vi "Combination_Digitizer_Driver_CLEANUP.vi"(0 "Mode":T1(ring), 1 "Horizontal Settings":T2={"number of records"=1, "reference position"=50.0, "min record length"=50000, "min sample rate"=200000.0, "enforce realtime"=FALSE, "maximum input frequency"=0.0} {"maximum input frequency" format="%.2f"; "min sample rate" step=1000000.0 format="%.0p"; "reference position" format="%.1f"; "number of records" step=1}, 2 "Vertical Settings":T4={"vertical coupling"=enum."DC", "probe attenuation"=20.0, "vertical range"=120.0, "vertical offset"=0.0} {"vertical offset" format="%.4f"; "vertical range" format="%.2f"; "probe attenuation" format="%.1f"}, 3 "Trigger settings":T3={"trigger level"=30.0, "trigger type"=enum."Edge", "Trigger Source"=enum."Channel 0", "Trigger Slope"=enum."Positive"} {"trigger level" format="%.2f"}, 5 "Channel Name":string="0", 11 "error in":errorcluster) -> (6 "Waveform Array":waveform(dbl)[](array[waveform]), 8 "Ch1_Plot":dbl[](array[numeric]), 15 "error out":errorcluster)   [LabVIEW 2010]
uses:
  <instrlib>/niScope/Acquire/niScope Multi Read Cluster.vi
  <instrlib>/niScope/Configure/Trigger/niScope Configure Trigger Edge.vi
  <instrlib>/niScope/Configure/Trigger/niScope Configure Trigger Digital.vi
  <instrlib>/niScope/Configure/Trigger/niScope Configure Trigger Immediate.vi
  <instrlib>/niScope/Controls/niScope trigger source.ctl
  <instrlib>/niScope/Controls/niScope trigger slope.ctl
  <instrlib>/niScope/Controls/niScope trigger source digital.ctl
  <instrlib>/niScope/Acquire/Fetch/niScope Multi Fetch Cluster.vi
  <instrlib>/niScope/Controls/niScope exportable signals.ctl
  <instrlib>/niScope/Controls/niScope export destinations.ctl
panel:
  out "Waveform":T5(graph)
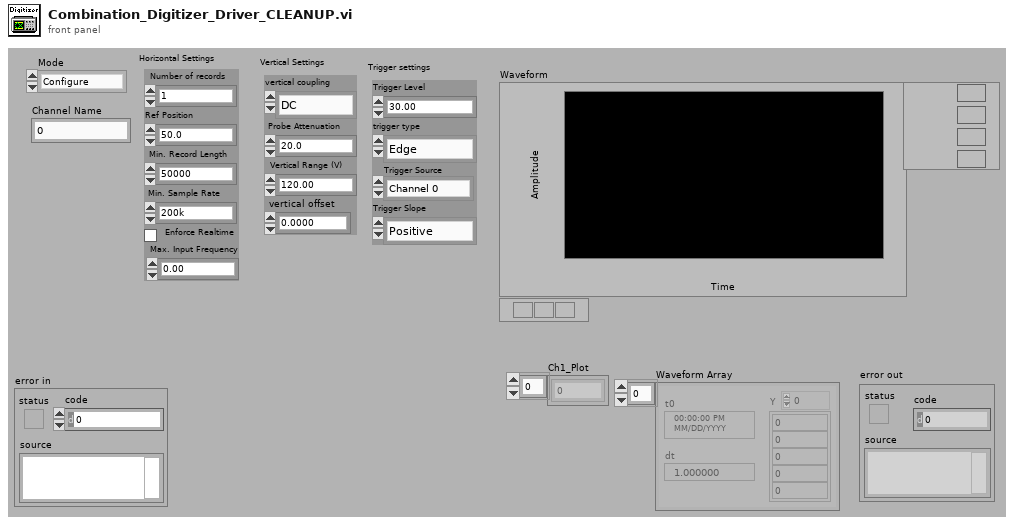
[diagram p1: front panel]
types:
  T1 = enum16{"Configure", "Read", "TriggerRead", "Close", "Init"}
  T2 = cluster{"number of records":i32, "reference position":dbl, "min record length":i32, "min sample rate":dbl, "enforce realtime":bool, "maximum input frequency":dbl}
  T3 = cluster{"trigger level":dbl, "trigger type":enum16{"Edge", "Digital", "Immediate"}, "Trigger Source":enum8{"Immediate", "Channel 0", "Channel 1", "Channel 2", "Channel 3", "Channel 4", "Channel 5", "Channel 6", "Channel 7", "External TRIG", "Software Trigger", "RTSI 0", "RTSI 1", "RTSI 2", "RTSI 3", "RTSI 4", "RTSI 5", "RTSI 6", "PFI 0", "PFI 1", "PFI 2", "PXI Star Trigger"}, "Trigger Slope":enum16{"Positive", "Negative"}}
  T4 = cluster{"vertical coupling":enum16{"AC", "DC", "Ground"}, "probe attenuation":dbl, "vertical range":dbl, "vertical offset":dbl}
  T5 = cluster{"relativeInitialX":dbl, "xIncrement":dbl, "wfm":dbl[]}[]
  T6 = typedef "niScope trigger source.ctl" = string
  T7 = typedef "niScope trigger source digital.ctl" = string
  T8 = typedef "niScope export destinations.ctl" = string
  T9 = cluster{"Dig1 Channels":string, "Channel1 Scale":dbl, "Dig1 Used":bool, "Dig1 Ref":refnum<k15>, "min record length":i32, "Dig2 Channels":string, "Dig2 Used":bool, "Dig2 Ref":refnum<k15>, "trigger type":enum16{"Edge", "Digital", "Immediate"}, "Vertical Settings":cluster{"vertical coupling":enum16{"AC", "DC", "Ground"}, "probe attenuation":dbl, "vertical range":dbl, "vertical offset":dbl}, "Horizontal Settings":cluster{"number of records":i32, "reference position":dbl, "min record length":i32, "min sample rate":dbl, "enforce realtime":bool, "maximum input frequency":dbl}, "Trigger settings":cluster{"trigger level":dbl, "trigger type":enum16{"Edge", "Digital", "Immediate"}, "Trigger Source":enum8{"Immediate", "Channel 0", "Channel 1", "Channel 2", "Channel 3", "Channel 4", "Channel 5", "Channel 6", "Channel 7", "External TRIG", "Software Trigger", "RTSI 0", "RTSI 1", "RTSI 2", "RTSI 3", "RTSI 4", "RTSI 5", "RTSI 6", "PFI 0", "PFI 1", "PFI 2", "PXI Star Trigger"}, "Trigger Slope":enum16{"Positive", "Negative"}}}
  T10 = enum8{"Immediate", "Channel 0", "Channel 1", "Channel 2", "Channel 3", "Channel 4", "Channel 5", "Channel 6", "Channel 7", "External TRIG", "Software Trigger", "RTSI 0", "RTSI 1", "RTSI 2", "RTSI 3", "RTSI 4", "RTSI 5", "RTSI 6", "PFI 0", "PFI 1", "PFI 2", "PXI Star Trigger"}
  T11 = typedef "niScope trigger slope.ctl" = i32
  T12 = typedef "niScope exportable signals.ctl" = u16
  T13 = cluster{"relativeInitialX":dbl, "xIncrement":dbl, "wfm":dbl[]}
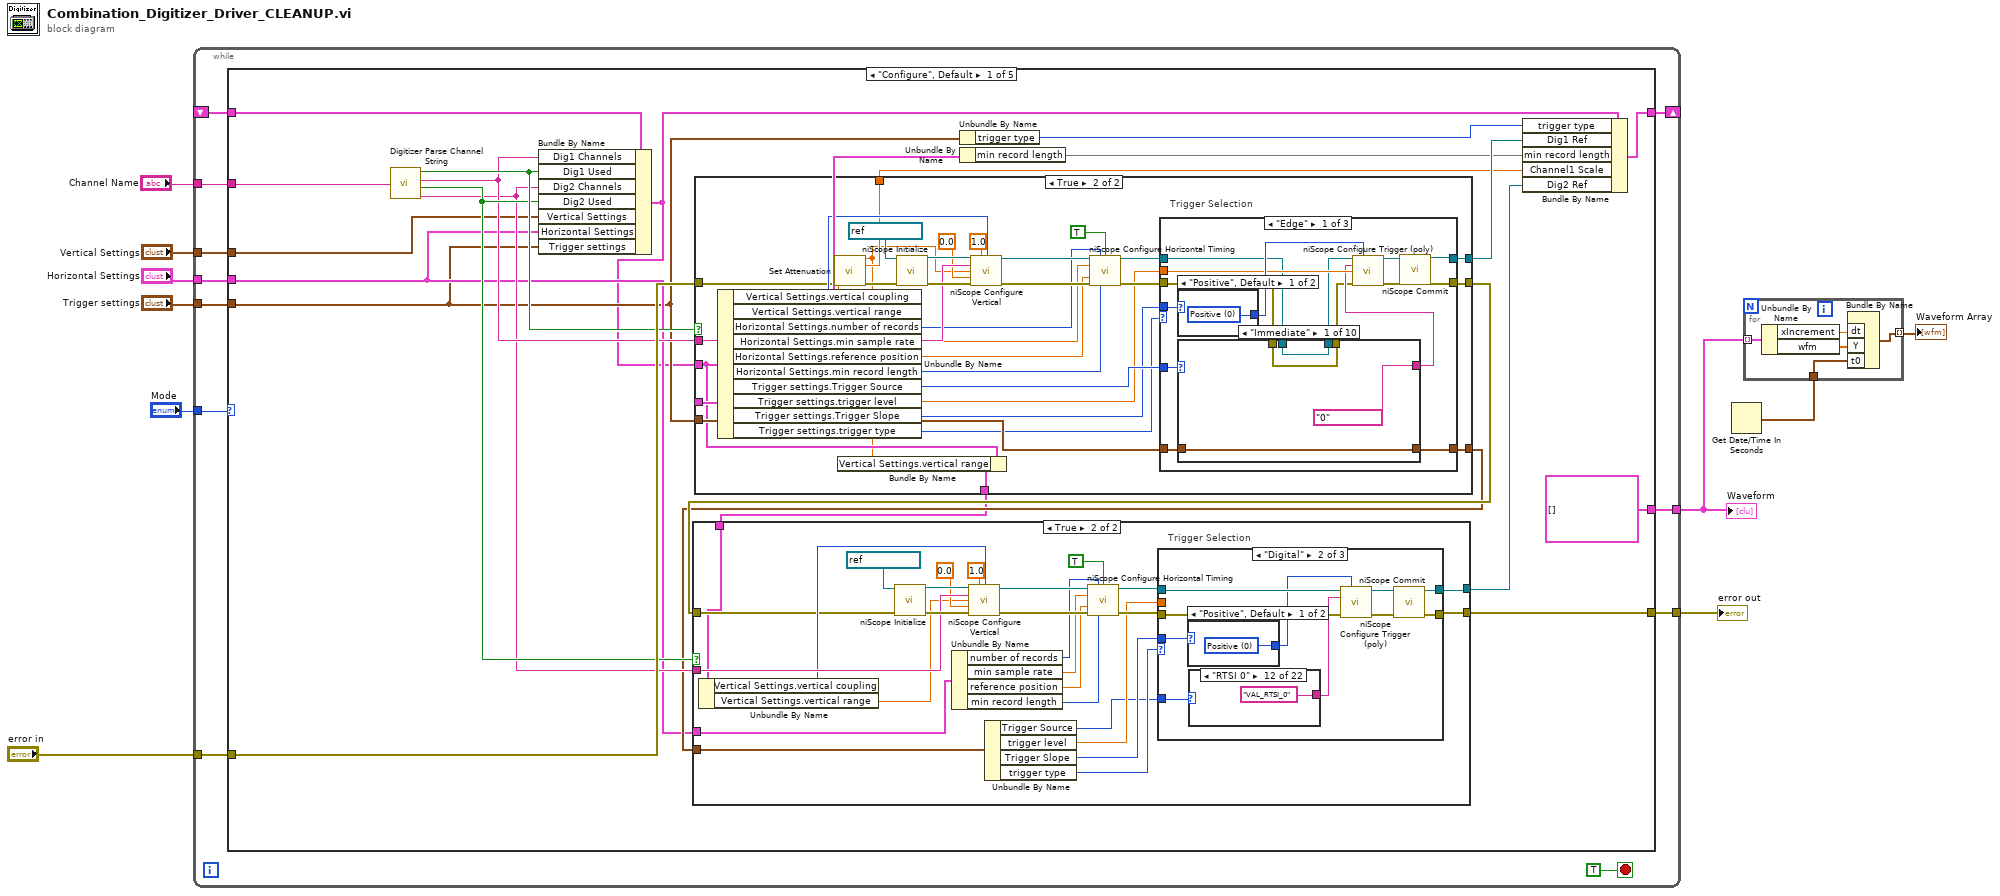
[diagram p0: block diagram]
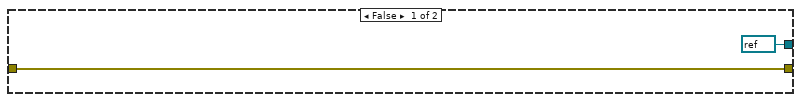
[diagram p2: hidden frame]
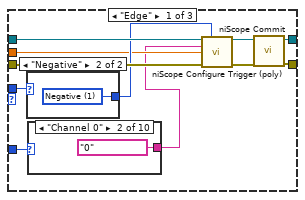
[diagram p3: hidden frame]
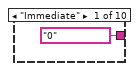
[diagram p4: hidden frame]
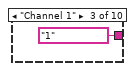
[diagram p5: hidden frame]
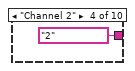
[diagram p6: hidden frame]
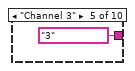
[diagram p7: hidden frame]
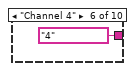
[diagram p8: hidden frame]
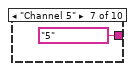
[diagram p9: hidden frame]
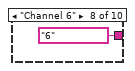
[diagram p10: hidden frame]
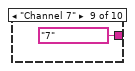
[diagram p11: hidden frame]
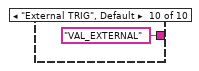
[diagram p12: hidden frame]
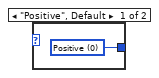
[diagram p13: hidden frame]
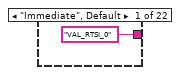
[diagram p14: hidden frame]
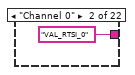
[diagram p15: hidden frame]
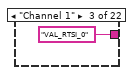
[diagram p16: hidden frame]
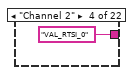
[diagram p17: hidden frame]
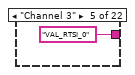
[diagram p18: hidden frame]
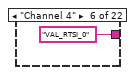
[diagram p19: hidden frame]
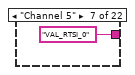
[diagram p20: hidden frame]
diagram:
  n1 = while {
    tunnel: "Mode" -> [w20]
    shift-right: [w14] -> _
    shift-left: _ -> [w19]
    tunnel: "error in" -> [w13]
    tunnel: "Channel Name" -> [w18]
    tunnel: "Vertical Settings" -> [w17]
    tunnel: "Horizontal Settings" -> [w16]
    tunnel: "Trigger settings" -> [w15]
    tunnel: [w12] -> w5
    tunnel: [w11] -> w3
    stop <- TRUE stop-if-true
    n2 = case shown="\"Configure\", Default" w20 {
      tunnel: w19 -> [w40 w280 w383 w410 w459]
      tunnel: w18 -> [w43 _ _ _ _]
      tunnel: w17 -> [w26 _ _ _ _]
      tunnel: w16 -> [w25 _ _ _ _]
      tunnel: w15 -> [w24 _ _ _ _]
      tunnel: [w42 w280 w383 w410 T9 {"Dig1 Channels"="", "Channel1 Scale"=0.0, "Dig1 Used"=FALSE, "Dig1 Ref"="", "min record length"=0, "Dig2 Channels"="", "Dig2 Used"=FALSE, "Dig2 Ref"="", "trigger type"=enum."Immediate", "Vertical Settings"={"vertical coupling"=enum."DC", "probe attenuation"=20.0, "vertical range"=120.0, "vertical offset"=0.0}, "Horizontal Settings"={"number of records"=1, "reference position"=50.0, "min record length"=50000, "min sample rate"=200000.0, "enforce realtime"=FALSE, "maximum input frequency"=0.0}, "Trigger settings"={"trigger level"=30.0, "trigger type"=enum."Edge", "Trigger Source"=enum."Channel 0", "Trigger Slope"=enum."Positive"}}] -> w14
      tunnel: w13 -> [w41 w286 w386 w416 w462]
      tunnel: [w36 w291 w389 w421 w465] -> w12
      tunnel: [T5 [] w278 T5 [] w409 T5 []] -> w11
      frame "Configure", Default {
        n3 = call "Digitizer Parse Channel String.vi"("Channel List"=w43) -> ("Dig2 Channels"=w32:string, "Dig2 Used?"=w34:bool, "Dig1 Channels"=w33:string, "Dig1 Used?"=w35:bool)
        n4 = Bundle By Name(cluster=w40, "Dig1 Channels"=w33, "Dig1 Used"=w35, "Dig2 Channels"=w32, "Dig2 Used"=w34, "Vertical Settings"=w26, "Horizontal Settings"=w25, "Trigger settings"=w24) -> (w23:T9)
        n5 = case shown="True" w35 {
          tunnel: [w139 w166] -> w44
          tunnel: w41 -> [w139 w160]
          tunnel: w33 -> [_ w164]
          tunnel: w23 -> [w135 w150]
          tunnel: [_ _] -> w22
          tunnel: w24 -> [w136 w152]
          tunnel: [refnum<k15> refnum ("instrument handle out") w155] -> w39
          tunnel: [1.0 ("Gain Multiplier") w153] -> w37
          tunnel: [w136 w151] -> w28
          tunnel: [w135 w148] -> w27
          frame False {
          }
          frame True {
            n6 = Unbundle By Name(w150) -> ("Vertical Settings.vertical coupling"=w163:enum16{"AC", "DC", "Ground"}, "Vertical Settings.vertical range"=w161:dbl, "Horizontal Settings.number of records"=w147:i32, "Horizontal Settings.min sample rate"=w146:dbl, "Horizontal Settings.reference position"=w145:dbl, "Horizontal Settings.min record length"=w144:i32, "Trigger settings.Trigger Source"=w143:T10, "Trigger settings.trigger level"=w142:dbl, "Trigger settings.Trigger Slope"=w141:enum16{"Positive", "Negative"}, "Trigger settings.trigger type"=w140:enum16{"Edge", "Digital", "Immediate"})
            n7 = call "Set Attenuation.vi"("vertical range"=w161, "error in"=w160) -> ("Requested Range"=w149:dbl, "Gain Multiplier"=w153:dbl, "error out"=w159:errorcluster)  [unwired: 11 in]
            n8 = Bundle By Name(cluster=w150, "Vertical Settings.vertical range"=w149) -> (w148:T9)
            n9 = call <instrlib>:"niScope Initialize.vi"("resource name"=refnum<k15> "PXI1Slot6", "error in"=w159) -> ("instrument handle"=w170:refnum<k15>, "error out"=w167:errorcluster)  [unwired: 12 in]
            n10 = call <instrlib>:"niScope Configure Vertical.vi"("instrument handle"=w170, "probe attenuation"=1.0, "vertical coupling"=w163, "channels"=w164, "vertical range"=w149, "vertical offset"=0.0, "error in"=w167) -> ("instrument handle out"=w157:refnum<k15>, "error out"=w156:errorcluster)  [unwired: 7 in]
            n11 = call <instrlib>:"niScope Configure Horizontal Timing.vi"("instrument handle"=w157, "number of records"=w147, "enforce realtime"=TRUE, "min sample rate"=w146, "reference position"=w145, "error in"=w156, "min record length"=w144) -> ("instrument handle out"=w168:refnum<k15>, "error out"=w169:errorcluster)  [unwired: 7 in]
            n12 = case "Trigger Selection" shown="\"Edge\"" w140 {
              tunnel: w169 -> [w172 w244 w273]
              tunnel: [w177 w237 w270] -> w166
              tunnel: w168 -> [w174 w243 w272]
              tunnel: [w178 w238 w271] -> w155
              tunnel: w143 -> [w182 w240 _]
              tunnel: w142 -> [w183 _ _]
              tunnel: w141 -> [w185 w242 _]
              tunnel: w152 -> [w176 w236 w269]
              tunnel: [w175 w236 w269] -> w151
              frame "Edge" {
                n13 = case shown="\"Positive\", Default" w185 {
                  tunnel: [w234 w235] -> w184
                  frame "Positive", Default {
                    w234 = T11 0 items=["Positive", "Negative"] ("trigger slope")
                  }
                  frame "Negative" {
                    w235 = T11 1 items=["Positive", "Negative"] ("trigger slope")
                  }
                }
                n14 = case shown="\"Immediate\"" w182 {
                  tunnel: [T6 "0" ("trigger source") T6 "0" ("trigger source") T6 "1" ("trigger source") T6 "2" ("trigger source") T6 "3" ("trigger source") T6 "4" ("trigger source") T6 "5" ("trigger source") T6 "6" ("trigger source") T6 "7" ("trigger source") T6 "VAL_EXTERNAL" ("trigger source")] -> w181
                  tunnel: w176 -> [w188 _ _ w208 w212 w216 w220 w224 w228 w232]
                  tunnel: [w188 T3 {"trigger level"=0.0, "trigger type"=enum."Digital", "Trigger Source"=enum."RTSI 0", "Trigger Slope"=enum."Positive"} ("Trigger settings") T3 {"trigger level"=0.0, "trigger type"=enum."Digital", "Trigger Source"=enum."RTSI 0", "Trigger Slope"=enum."Positive"} ("Trigger settings") w208 w212 w216 w220 w224 w228 w232] -> w175
                  tunnel: w174 -> [w187 w193 w201 w207 w211 w215 w219 w223 w227 w231]
                  tunnel: [w187 w191 w200 w207 w211 w215 w219 w223 w227 w231] -> w173
                  tunnel: w172 -> [w186 w192 w199 w206 w210 w214 w218 w222 w226 w230]
                  tunnel: [w186 w190 w198 w206 w210 w214 w218 w222 w226 w230] -> w171
                  frame "Immediate" {
                  }
                  frame "Channel 0" {
                    w194 = T12 1 items=["None"=0, "Start Trigger"=2, "Advance Trigger"=5, "Reference Trigger"=1, "End of Record Event"=4, "End of Acquisition Event"=3, "Ready for Start Event"=7, "Ready for Advance Event"=6, "Ready for Reference Event"=10, "Reference Clock"=100, "Sample Clock"=101, "5 Volt Power"=13] ("signal")
                    n15 = call <instrlib>:"niScope Export Signal.vi"("instrument handle"=w193, "signal"=w194, "output terminal"=T8 "VAL_RTSI_0", "error in"=w192) -> ("instrument handle out"=w191:refnum<k15>, "error out"=w190:errorcluster)  [unwired: 10 in]
                  }
                  frame "Channel 1" {
                    w202 = T12 1 items=["None"=0, "Start Trigger"=2, "Advance Trigger"=5, "Reference Trigger"=1, "End of Record Event"=4, "End of Acquisition Event"=3, "Ready for Start Event"=7, "Ready for Advance Event"=6, "Ready for Reference Event"=10, "Reference Clock"=100, "Sample Clock"=101, "5 Volt Power"=13] ("signal")
                    n16 = call <instrlib>:"niScope Export Signal.vi"("instrument handle"=w201, "signal"=w202, "output terminal"=T8 "VAL_RTSI_0", "error in"=w199) -> ("instrument handle out"=w200:refnum<k15>, "error out"=w198:errorcluster)  [unwired: 10 in]
                  }
                  frame "Channel 2" {
                  }
                  frame "Channel 3" {
                  }
                  frame "Channel 4" {
                  }
                  frame "Channel 5" {
                  }
                  frame "Channel 6" {
                  }
                  frame "Channel 7" {
                  }
                  frame "External TRIG", Default {
                  }
                }
                n17 = call-poly <instrlib>:"niScope Configure Trigger (poly).vi"("instrument handle"=w173, "trigger slope"=w184, "trigger source"=w181, "trigger level"=w183, "error in"=w171) -> ("instrument handle out"=w180:refnum<k15>, "error out"=w179:errorcluster)  [unwired: 9 in]
                n18 = call <instrlib>:"niScope Commit.vi"("instrument handle"=w180, "error in"=w179) -> ("instrument handle out"=w178:refnum<k15>, "error out"=w177:errorcluster)  [unwired: 12 in]
              }
              frame "Digital" {
                n19 = case shown="\"Negative\"" w242 {
                  tunnel: [w267 w268] -> w241
                  frame "Positive", Default {
                    w267 = T11 0 items=["Positive", "Negative"] ("trigger slope")
                  }
                  frame "Negative" {
                    w268 = T11 1 items=["Positive", "Negative"] ("trigger slope")
                  }
                }
                n20 = case shown="\"PXI Star Trigger\"" w240 {
                  tunnel: [T7 "VAL_RTSI_0" ("trigger source") T7 "VAL_RTSI_0" ("trigger source") T7 "VAL_RTSI_0" ("trigger source") T7 "VAL_RTSI_0" ("trigger source") T7 "VAL_RTSI_0" ("trigger source") T7 "VAL_RTSI_0" ("trigger source") T7 "VAL_RTSI_0" ("trigger source") T7 "VAL_RTSI_0" ("trigger source") T7 "VAL_RTSI_0" ("trigger source") T7 "VAL_RTSI_0" ("trigger source") T7 "VAL_RTSI_0" ("trigger source") T7 "VAL_RTSI_0" ("trigger source") T7 "VAL_RTSI_1" ("trigger source") T7 "VAL_RTSI_2" ("trigger source") T7 "VAL_RTSI_3" ("trigger source") T7 "VAL_RTSI_4" ("trigger source") T7 "VAL_RTSI_5" ("trigger source") T7 "VAL_RTSI_6" ("trigger source") T7 "VAL_PFI_0" ("trigger source") T7 "VAL_PFI_1" ("trigger source") T7 "VAL_PFI_2" ("trigger source") T7 "VAL_PXI_STAR" ("trigger source")] -> w239
                  frame "Immediate", Default {
                  }
                  frame "Channel 0" {
                  }
                  frame "Channel 1" {
                  }
                  frame "Channel 2" {
                  }
                  frame "Channel 3" {
                  }
                  frame "Channel 4" {
                  }
                  frame "Channel 5" {
                  }
                  frame "Channel 6" {
                  }
                  frame "Channel 7" {
                  }
                  frame "External TRIG" {
                  }
                  frame "Software Trigger" {
                  }
                  frame "RTSI 0" {
                  }
                  frame "RTSI 1" {
                  }
                  frame "RTSI 2" {
                  }
                  frame "RTSI 3" {
                  }
                  frame "RTSI 4" {
                  }
                  frame "RTSI 5" {
                  }
                  frame "RTSI 6" {
                  }
                  frame "PFI 0" {
                  }
                  frame "PFI 1" {
                  }
                  frame "PFI 2" {
                  }
                  frame "PXI Star Trigger" {
                  }
                }
                n21 = call-poly <instrlib>:"niScope Configure Trigger (poly).vi"("instrument handle"=w243, "trigger slope"=w241, "trigger source"=w239, "error in"=w244) -> ("instrument handle out"=w238:refnum<k15>, "error out"=w237:errorcluster)  [unwired: 10 in]
              }
              frame "Immediate", Default {
                n22 = call-poly <instrlib>:"niScope Configure Trigger (poly).vi"("instrument handle"=w272, "error in"=w273) -> ("instrument handle out"=w271:refnum<k15>, "error out"=w270:errorcluster)  [unwired: 12 in]
              }
            }
          }
        }
        n23 = case shown="True" w34 {
          tunnel: [w46 w53] -> w36
          tunnel: w44 -> [w46 w58]
          tunnel: w32 -> [_ w70]
          tunnel: w25 -> [_ w64]
          tunnel: w28 -> [_ w59]
          tunnel: [refnum<k15> refnum ("instrument handle out") w54] -> w38
          tunnel: w27 -> [_ w47]
          frame False {
          }
          frame True {
            n24 = Unbundle By Name(w47) -> ("Vertical Settings.vertical coupling"=w69:enum16{"AC", "DC", "Ground"}, "Vertical Settings.vertical range"=w57:dbl)
            n25 = call <instrlib>:"niScope Initialize.vi"("resource name"=refnum<k15> "PXI1Slot4", "error in"=w58) -> ("instrument handle"=w73:refnum<k15>, "error out"=w72:errorcluster)  [unwired: 12 in]
            n26 = Unbundle By Name(w64) -> ("number of records"=w63:i32, "min sample rate"=w62:dbl, "reference position"=w61:dbl, "min record length"=w60:i32)
            n27 = call <instrlib>:"niScope Configure Vertical.vi"("instrument handle"=w73, "probe attenuation"=1.0, "vertical coupling"=w69, "channels"=w70, "vertical range"=w57, "vertical offset"=0.0, "error in"=w72) -> ("instrument handle out"=w66:refnum<k15>, "error out"=w65:errorcluster)  [unwired: 7 in]
            n28 = Unbundle By Name(w59) -> ("Trigger Source"=w48:T10, "trigger level"=w51:dbl, "Trigger Slope"=w49:enum16{"Positive", "Negative"}, "trigger type"=w50:enum16{"Edge", "Digital", "Immediate"})
            n29 = call <instrlib>:"niScope Configure Horizontal Timing.vi"("instrument handle"=w66, "number of records"=w63, "enforce realtime"=TRUE, "min sample rate"=w62, "reference position"=w61, "error in"=w65, "min record length"=w60) -> ("instrument handle out"=w55:refnum<k15>, "error out"=w52:errorcluster)  [unwired: 7 in]
            n30 = case "Trigger Selection" shown="\"Digital\"" w50 {
              tunnel: w52 -> [w84 w106 w134]
              tunnel: [w74 w97 w131] -> w53
              tunnel: w55 -> [w83 w105 w133]
              tunnel: [w76 w98 w132] -> w54
              tunnel: w48 -> [w79 w102 _]
              tunnel: w51 -> [w80 _ _]
              tunnel: w49 -> [w82 w104 _]
              frame "Edge" {
                n31 = case shown="\"Negative\"" w82 {
                  tunnel: [w95 w96] -> w81
                  frame "Positive", Default {
                    w95 = T11 0 items=["Positive", "Negative"] ("trigger slope")
                  }
                  frame "Negative" {
                    w96 = T11 1 items=["Positive", "Negative"] ("trigger slope")
                  }
                }
                n32 = case shown="\"Channel 0\"" w79 {
                  tunnel: [T6 "0" ("trigger source") T6 "0" ("trigger source") T6 "1" ("trigger source") T6 "2" ("trigger source") T6 "3" ("trigger source") T6 "4" ("trigger source") T6 "5" ("trigger source") T6 "6" ("trigger source") T6 "7" ("trigger source") T6 "VAL_EXTERNAL" ("trigger source")] -> w78
                  frame "Immediate" {
                  }
                  frame "Channel 0" {
                  }
                  frame "Channel 1" {
                  }
                  frame "Channel 2" {
                  }
                  frame "Channel 3" {
                  }
                  frame "Channel 4" {
                  }
                  frame "Channel 5" {
                  }
                  frame "Channel 6" {
                  }
                  frame "Channel 7" {
                  }
                  frame "External TRIG", Default {
                  }
                }
                n33 = call-poly <instrlib>:"niScope Configure Trigger (poly).vi"("instrument handle"=w83, "trigger slope"=w81, "trigger source"=w78, "trigger level"=w80, "error in"=w84) -> ("instrument handle out"=w77:refnum<k15>, "error out"=w75:errorcluster)  [unwired: 9 in]
                n34 = call <instrlib>:"niScope Commit.vi"("instrument handle"=w77, "error in"=w75) -> ("instrument handle out"=w76:refnum<k15>, "error out"=w74:errorcluster)  [unwired: 12 in]
              }
              frame "Digital" {
                n35 = case shown="\"Positive\", Default" w104 {
                  tunnel: [w129 w130] -> w103
                  frame "Positive", Default {
                    w129 = T11 0 items=["Positive", "Negative"] ("trigger slope")
                  }
                  frame "Negative" {
                    w130 = T11 1 items=["Positive", "Negative"] ("trigger slope")
                  }
                }
                n36 = case shown="\"RTSI 0\"" w102 {
                  tunnel: [T7 "VAL_RTSI_0" ("trigger source") T7 "VAL_RTSI_0" ("trigger source") T7 "VAL_RTSI_0" ("trigger source") T7 "VAL_RTSI_0" ("trigger source") T7 "VAL_RTSI_0" ("trigger source") T7 "VAL_RTSI_0" ("trigger source") T7 "VAL_RTSI_0" ("trigger source") T7 "VAL_RTSI_0" ("trigger source") T7 "VAL_RTSI_0" ("trigger source") T7 "VAL_RTSI_0" ("trigger source") T7 "VAL_RTSI_0" ("trigger source") T7 "VAL_RTSI_0" ("trigger source") T7 "VAL_RTSI_1" ("trigger source") T7 "VAL_RTSI_2" ("trigger source") T7 "VAL_RTSI_3" ("trigger source") T7 "VAL_RTSI_4" ("trigger source") T7 "VAL_RTSI_5" ("trigger source") T7 "VAL_RTSI_6" ("trigger source") T7 "VAL_PFI_0" ("trigger source") T7 "VAL_PFI_1" ("trigger source") T7 "VAL_PFI_2" ("trigger source") T7 "VAL_PXI_STAR" ("trigger source")] -> w101
                  frame "Immediate", Default {
                  }
                  frame "Channel 0" {
                  }
                  frame "Channel 1" {
                  }
                  frame "Channel 2" {
                  }
                  frame "Channel 3" {
                  }
                  frame "Channel 4" {
                  }
                  frame "Channel 5" {
                  }
                  frame "Channel 6" {
                  }
                  frame "Channel 7" {
                  }
                  frame "External TRIG" {
                  }
                  frame "Software Trigger" {
                  }
                  frame "RTSI 0" {
                  }
                  frame "RTSI 1" {
                  }
                  frame "RTSI 2" {
                  }
                  frame "RTSI 3" {
                  }
                  frame "RTSI 4" {
                  }
                  frame "RTSI 5" {
                  }
                  frame "RTSI 6" {
                  }
                  frame "PFI 0" {
                  }
                  frame "PFI 1" {
                  }
                  frame "PFI 2" {
                  }
                  frame "PXI Star Trigger" {
                  }
                }
                n37 = call-poly <instrlib>:"niScope Configure Trigger (poly).vi"("instrument handle"=w105, "trigger slope"=w103, "trigger source"=w101, "error in"=w106) -> ("instrument handle out"=w100:refnum<k15>, "error out"=w99:errorcluster)  [unwired: 10 in]
                n38 = call <instrlib>:"niScope Commit.vi"("instrument handle"=w100, "error in"=w99) -> ("instrument handle out"=w98:refnum<k15>, "error out"=w97:errorcluster)  [unwired: 12 in]
              }
              frame "Immediate", Default {
                n39 = call-poly <instrlib>:"niScope Configure Trigger (poly).vi"("instrument handle"=w133, "error in"=w134) -> ("instrument handle out"=w132:refnum<k15>, "error out"=w131:errorcluster)  [unwired: 12 in]
              }
            }
          }
        }
        n40 = Unbundle By Name(w24) -> ("trigger type"=w29:enum16{"Edge", "Digital", "Immediate"})
        n41 = Unbundle By Name(w22) -> ("min record length"=w31)
        n42 = Bundle By Name(cluster=w23, "trigger type"=w29, "Dig1 Ref"=w39, "min record length"=w31, "Channel1 Scale"=w37, "Dig2 Ref"=w38) -> (w42:T9)
      }
      frame "Read" {
        n43 = Unbundle By Name(w280) -> ("trigger type"=w275:enum16{"Edge", "Digital", "Immediate"}, "Dig1 Used"=w290:bool, "Dig1 Ref"=w289:refnum<k15>, "Dig1 Channels"=w288:string, "min record length"=w287:i32, "Channel1 Scale"=w281:dbl)
        n44 = Unbundle By Name(w280) -> ("trigger type"=w274:enum16{"Edge", "Digital", "Immediate"}, "Dig2 Used"=w285:bool, "Dig2 Ref"=w284:refnum<k15>, "Dig2 Channels"=w283:string, "min record length"=w282:i32)
        n45 = case shown="True" w290 {
          tunnel: w288 -> [_ w354]
          tunnel: w286 -> [w348 w352]
          tunnel: w289 -> [_ w355]
          tunnel: [w348 w350] -> w292
          tunnel: [T5 [] ("waveform") w351] -> w293
          tunnel: w287 -> [_ w353]
          tunnel: w275 -> [_ w349]
          frame False {
          }
          frame True {
            n46 = case shown="\"Digital\", Default" w349 {
              tunnel: w355 -> [w362 w372]
              tunnel: w354 -> [w361 w371]
              tunnel: w353 -> [w360 w370]
              tunnel: w352 -> [w359 w369]
              tunnel: [w357 w364] -> w351
              tunnel: [w356 w367] -> w350
              frame "Immediate" {
                n47 = call-poly <instrlib>:"niScope Read (poly).vi"("timeout"=10.0, "error in"=w359, "numSamples"=w360, "channels"=w361, "instrument handle"=w362) -> ("error out"=w356:errorcluster, "waveform"=w357:T5)  [unwired: 3 in, 2 out]
              }
              frame "Digital", Default {
                n48 = call-poly <instrlib>:"niScope Fetch (poly).vi"("timeout"=10.0, "error in"=w369, "numSamples"=w370, "channels"=w371, "instrument handle"=w372) -> ("error out"=w366:errorcluster, "waveform"=w365:T5, "instrument handle out"=w363:refnum<k15>)  [unwired: 3 in, 1 out]
                n49 = case shown="Error" w366 {
                  tunnel: w366 -> [w373 w379]
                  tunnel: [w373 w376] -> w367
                  tunnel: w365 -> [w374 _]
                  tunnel: [w374 T5 [{"relativeInitialX"=0.0, "xIncrement"=0.0, "wfm"=[]}, {"relativeInitialX"=0.0, "xIncrement"=0.0, "wfm"=[]}] ("waveform")] -> w364
                  tunnel: w363 -> [_ w375]
                  frame No Error {
                  }
                  frame Error {
                    n50 = call <vilib>:"Clear Errors.vi"("error in (no error)"=w379) -> ("error out"=w377:errorcluster)  [unwired: 6 in]
                    n51 = call <instrlib>:"niScope Abort.vi"("instrument handle"=w375, "error in"=w377) -> ("error out"=w376:errorcluster)  [unwired: 12 in, 1 out]
                  }
                }
              }
            }
          }
        }
        n52 = case shown="True" w285 {
          tunnel: w283 -> [_ w319]
          tunnel: w292 -> [w315 w317]
          tunnel: w284 -> [_ w320]
          tunnel: w282 -> [_ w318]
          tunnel: [w315 w322] -> w291
          tunnel: [T5 [] ("waveform") w321] -> w296
          tunnel: w274 -> [_ w316]
          frame False {
          }
          frame True {
            n53 = case shown="\"Digital\", Default" w316 {
              tunnel: w320 -> [w329 w339]
              tunnel: w319 -> [w328 w338]
              tunnel: w318 -> [w327 w337]
              tunnel: w317 -> [w326 w336]
              tunnel: [w324 w332] -> w321
              tunnel: [w323 w333] -> w322
              frame "Immediate" {
                n54 = call-poly <instrlib>:"niScope Read (poly).vi"("timeout"=10.0, "error in"=w326, "numSamples"=w327, "channels"=w328, "instrument handle"=w329) -> ("error out"=w323:errorcluster, "waveform"=w324:T5)  [unwired: 3 in, 2 out]
              }
              frame "Digital", Default {
                n55 = call-poly <instrlib>:"niScope Fetch (poly).vi"("timeout"=10.0, "error in"=w336, "numSamples"=w337, "channels"=w338, "instrument handle"=w339) -> ("error out"=w331:errorcluster, "waveform"=w334:T5, "instrument handle out"=w330:refnum<k15>)  [unwired: 3 in, 1 out]
                n56 = case shown="Error" w331 {
                  tunnel: w331 -> [w340 w346]
                  tunnel: [w340 w342] -> w333
                  tunnel: w334 -> [w341 _]
                  tunnel: [w341 T5 [{"relativeInitialX"=0.0, "xIncrement"=0.0, "wfm"=[]}, {"relativeInitialX"=0.0, "xIncrement"=0.0, "wfm"=[]}] ("waveform")] -> w332
                  tunnel: w330 -> [_ w344]
                  frame No Error {
                  }
                  frame Error {
                    n57 = call <vilib>:"Clear Errors.vi"("error in (no error)"=w346) -> ("error out"=w343:errorcluster)  [unwired: 6 in]
                    n58 = call <instrlib>:"niScope Abort.vi"("instrument handle"=w344, "error in"=w343) -> ("error out"=w342:errorcluster)  [unwired: 12 in, 1 out]
                  }
                }
              }
            }
          }
        }
        n59 = Greater?(x=w281, y=1.0) -> (0:w295:bool)
        n60 = case shown="True" w295 {
          tunnel: w293 -> [w299 w313]
          tunnel: w281 -> [_ w300]
          tunnel: w296 -> [w298 w306]
          tunnel: [w297 w305] -> w278
          frame False {
            n61 = Build Array (concatenate)(w299, w298) -> (w297:T5)
          }
          frame True {
            # "Add scaling from TEGAM, if used"
            n62 = Index Array(array=w313, index #1=0 ("index"), index #2=1 ("index")) -> (element #1=w310:T13, element #2=w302:T13)
            n63 = Unbundle By Name(w310) -> ("wfm"=w312:dbl[])
            n64 = Unbundle By Name(w302) -> ("wfm"=w304:dbl[])
            n65 = Multiply(x=w312, y=w300) -> (x*y=w309:dbl[])
            n66 = Multiply(x=w304, y=w300) -> (x*y=w303:dbl[])
            n67 = Bundle By Name(cluster=w310, "wfm"=w309) -> (w307:T13)
            n68 = Bundle By Name(cluster=w302, "wfm"=w303) -> (w301:T13)
            n69 = Build Array (concatenate)(w307, w301, w306) -> (w305:T5)
          }
        }
        n70 = Index Array(array=w278, index=0) -> (element=w277:T13)
        n71 = Unbundle By Name(w277) -> ("wfm"=→"Ch1_Plot":dbl[])
      }
      frame "Init" {
        n72 = Unbundle By Name(w383) -> ("trigger type"=w382:enum16{"Edge", "Digital", "Immediate"}, "Dig1 Used"=w388:bool, "Dig1 Ref"=w387:refnum<k15>)
        n73 = Unbundle By Name(w383) -> ("trigger type"=w381:enum16{"Edge", "Digital", "Immediate"}, "Dig2 Used"=w385:bool, "Dig2 Ref"=w384:refnum<k15>)
        n74 = case shown="True" w388 {
          tunnel: w386 -> [w400 w403]
          tunnel: w387 -> [_ w404]
          tunnel: [w400 w402] -> w390
          tunnel: w382 -> [_ w401]
          frame False {
          }
          frame True {
            n75 = case shown="\"Digital\", Default" w401 {
              tunnel: w404 -> [_ w407]
              tunnel: w403 -> [w405 w406]
              tunnel: [w405 w408] -> w402
              frame "Immediate" {
              }
              frame "Digital", Default {
                n76 = call <instrlib>:"niScope Initiate Acquisition.vi"("instrument handle"=w407, "error in"=w406) -> ("error out"=w408:errorcluster)  [unwired: 12 in, 1 out]
              }
            }
          }
        }
        n77 = case shown="True" w385 {
          tunnel: w390 -> [w391 w393]
          tunnel: w384 -> [_ w394]
          tunnel: [w391 w395] -> w389
          tunnel: w381 -> [_ w392]
          frame False {
          }
          frame True {
            n78 = case shown="\"Digital\", Default" w392 {
              tunnel: w394 -> [_ w398]
              tunnel: w393 -> [w396 w397]
              tunnel: [w396 w399] -> w395
              frame "Immediate" {
              }
              frame "Digital", Default {
                n79 = call <instrlib>:"niScope Initiate Acquisition.vi"("instrument handle"=w398, "error in"=w397) -> ("error out"=w399:errorcluster)  [unwired: 12 in, 1 out]
              }
            }
          }
        }
      }
      frame "TriggerRead" {
        n80 = Unbundle By Name(w410) -> ("Dig1 Used"=w420:bool, "Dig1 Ref"=w419:refnum<k15>, "Dig1 Channels"=w418:string, "min record length"=w417:i32, "Channel1 Scale"=w411:dbl)
        n81 = Unbundle By Name(w410) -> ("Dig2 Used"=w415:bool, "Dig2 Ref"=w414:refnum<k15>, "Dig2 Channels"=w413:string, "min record length"=w412:i32)
        n82 = case shown="True" w420 {
          tunnel: w418 -> [_ w455]
          tunnel: w416 -> [w450 w456]
          tunnel: w419 -> [_ w454]
          tunnel: [w450 w451] -> w422
          tunnel: [T5 [] ("waveform") w453] -> w423
          tunnel: w417 -> [_ w452]
          frame False {
          }
          frame True {
            n83 = call-poly <instrlib>:"niScope Read (poly).vi"("error in"=w456, "numSamples"=w452, "channels"=w455, "instrument handle"=w454) -> ("error out"=w451:errorcluster, "waveform"=w453:T5)  [unwired: 4 in, 2 out]
          }
        }
        n84 = case shown="True" w415 {
          tunnel: w413 -> [_ w447]
          tunnel: w422 -> [w442 w448]
          tunnel: w414 -> [_ w446]
          tunnel: w412 -> [_ w445]
          tunnel: [w442 w443] -> w421
          tunnel: [T5 [] ("waveform") w444] -> w426
          frame False {
          }
          frame True {
            n85 = call-poly <instrlib>:"niScope Read (poly).vi"("error in"=w448, "numSamples"=w445, "channels"=w447, "instrument handle"=w446) -> ("error out"=w443:errorcluster, "waveform"=w444:T5)  [unwired: 4 in, 2 out]
          }
        }
        n86 = Greater?(x=w411, y=10.0) -> (0:w425:bool)
        n87 = case shown="True" w425 {
          tunnel: w423 -> [w429 w440]
          tunnel: w411 -> [_ w432]
          tunnel: w426 -> [w428 w431]
          tunnel: [w427 w430] -> w409
          frame False {
            n88 = Build Array (concatenate)(w429, w428) -> (w427:T5)
          }
          frame True {
            # "Add scaling from TEGAM, if used"
            n89 = Index Array(array=w440, index #1=0 ("index"), index #2=1 ("index")) -> (element #1=w437:T13, element #2=w434:T13)
            n90 = Unbundle By Name(w437) -> ("wfm"=w439:dbl[])
            n91 = Multiply(x=w439, y=w432) -> (x*y=w436:dbl[])
            n92 = Bundle By Name(cluster=w437, "wfm"=w436) -> (w433:T13)
            n93 = Build Array (concatenate)(w433, w434, w431) -> (w430:T5)
          }
        }
      }
      frame "Close" {
        n94 = Unbundle By Name(w459) -> ("Dig1 Used"=w464:bool, "Dig1 Ref"=w463:refnum<k15>)
        n95 = Unbundle By Name(w459) -> ("Dig2 Used"=w461:bool, "Dig2 Ref"=w460:refnum<k15>)
        n96 = case shown="True" w464 {
          tunnel: w462 -> [w471 w472]
          tunnel: w463 -> [_ w473]
          tunnel: [w471 w474] -> w466
          frame False {
          }
          frame True {
            n97 = call <instrlib>:"niScope Close.vi"("instrument handle"=w473, "error in"=w472) -> ("error out"=w474:errorcluster)  [unwired: 13 in]
          }
        }
        n98 = case shown="True" w461 {
          tunnel: w466 -> [w467 w469]
          tunnel: w460 -> [_ w468]
          tunnel: [w467 w470] -> w465
          frame False {
          }
          frame True {
            n99 = call <instrlib>:"niScope Close.vi"("instrument handle"=w468, "error in"=w469) -> ("error out"=w470:errorcluster)  [unwired: 13 in]
          }
        }
      }
    }
  }
  "error out" <- w5
  "Waveform" <- w3
  n100 = Get Date/Time In Seconds() -> (seconds since 1Jan1904=w1:timestamp)
  n101 = for {
    tunnel: w3 -> [w479] mode=indexing
    tunnel: [w476] -> w2 mode=indexing
    tunnel: w1 -> [w475]
    n102 = Unbundle By Name(w479) -> ("xIncrement"=w478:dbl, "wfm"=w477:dbl[])
    n103 = Bundle By Name("dt"=w478, "Y"=w477, "t0"=w475) -> (w476:waveform(dbl))  [unwired: 1 in]
  }
  "Waveform Array" <- w2
